vi "SRI8610C-DataFile Message Loop.vi"(7 "error in (no error)":errorcluster, 10 "Message Queues":T2) -> (0 "error out":errorcluster)   [LabVIEW 2020, in "SRI8610C-GasChromatograph.lvlib"]
uses:
  SRI8610C-GasChromatograph.lvlib
  support/Message Queue/All Message Queues.ctl
  support/Message Queue/Message Cluster.ctl
  SRI8160C/LabVIEW/Controls/SRI8610C-DataClusterV2.ctl
  SRI8160C/LabVIEW/Controls/SRI8610C-States-InitRun.ctl
  support/Message Queue/Enqueue Message (Single).vi
  support/Message Queue/Message Queue.lvlib
  Logging/Logging.lvlib
panel:
  out "Butane % Array":string[](array[string])
  out "GC Full Data Channels":T1[](array[typedef])
  out "Elapsed Time Since Last Update (sec)":dbl
  out "Numeric":i32
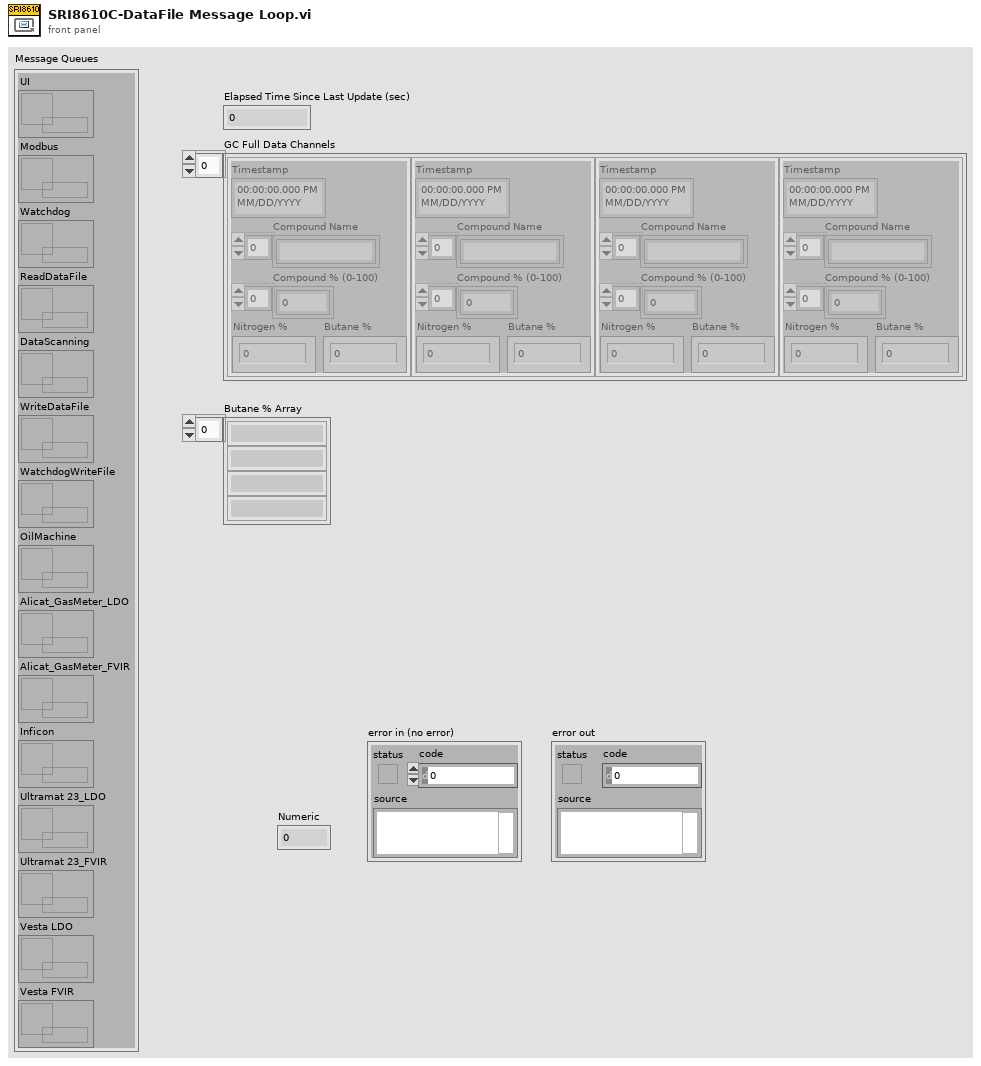
[diagram p1: front panel]
types:
  T1 = typedef "SRI8610C-DataClusterV2.ctl" = cluster{"Timestamp":timestamp, "Compound Name":string[], "Compound % (0-100)":dbl[], "Nitrogen %":dbl, "Butane %":dbl}
  T2 = typedef "Message Queue.lvlib/All Message Queues.ctl" = cluster{"UI":refnum<queue>, "Modbus":refnum<queue>, "Watchdog":refnum<queue>, "ReadDataFile":refnum<queue>, "DataScanning":refnum<queue>, "WriteDataFile":refnum<queue>, "WatchdogWriteFile":refnum<queue>, "OilMachine":refnum<queue>, "Alicat_GasMeter_LDO":refnum<queue>, "Inficon":refnum<queue>, "Ultramat 23_LDO":refnum<queue>, "Alicat_GasMeter_FVIR":refnum<queue>, "Ultramat 23_FVIR":refnum<queue>, "Vesta LDO":refnum<queue>, "Vesta FVIR":refnum<queue>}
  T3 = typedef "SRI8610C-States-InitRun.ctl" = enum16{"Initialize", "Run"}
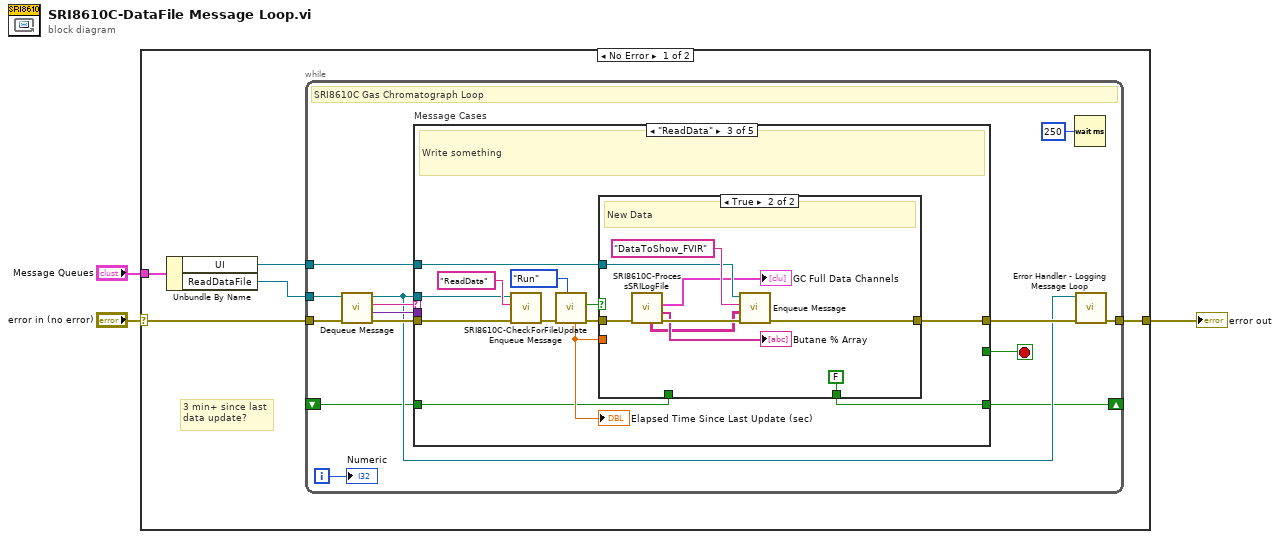
[diagram p0: block diagram]
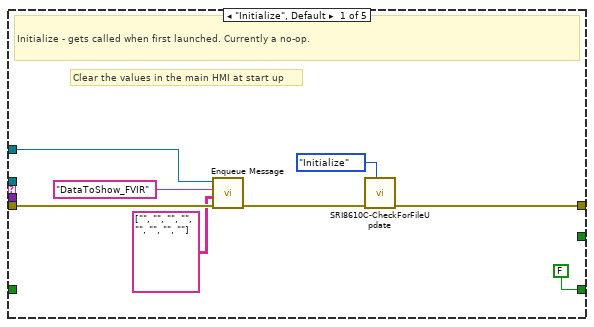
[diagram p2: hidden frame]
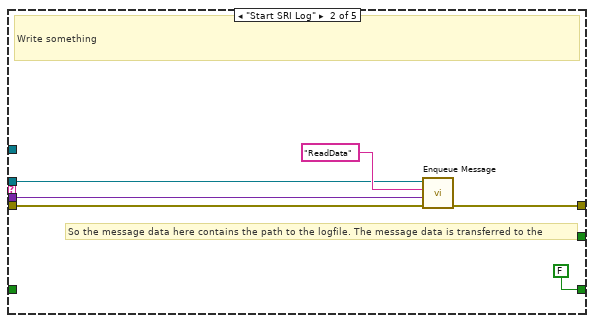
[diagram p3: hidden frame]
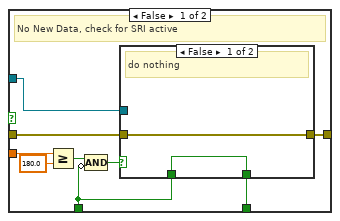
[diagram p4: hidden frame]
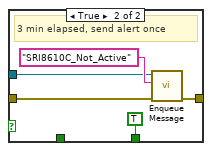
[diagram p5: hidden frame]
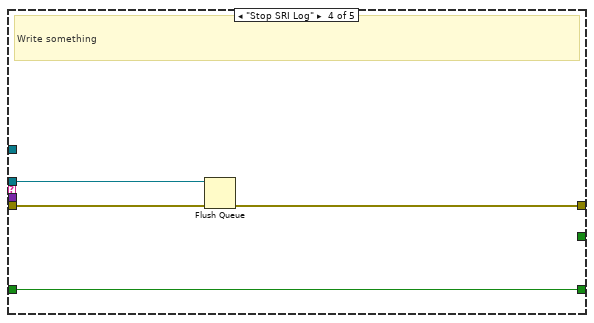
[diagram p6: hidden frame]
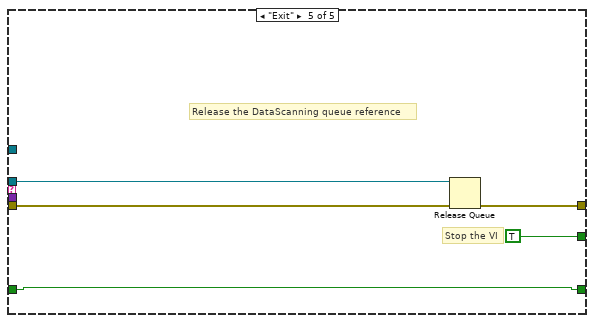
[diagram p7: hidden frame]
diagram:
  n1 = case shown="No Error" "error in (no error)" {
    selector: "error in (no error)" -> [w6 w82]
    tunnel: "Message Queues" -> [w8 _]
    tunnel: [w7 w82] -> w1
    frame No Error {
      # "3 min+ since last\ndata update?"
      n2 = Unbundle By Name(w8) -> ("UI"=w4:refnum<queue>, "ReadDataFile"=w5:refnum<queue>)
      n3 = while {
        tunnel: w5 -> [w17]
        tunnel: w6 -> [w21]
        tunnel: [w16] -> w7
        tunnel: w4 -> [w13]
        shift-right: [w9] -> _
        shift-left: _ -> [w10]
        i -> [w12]
        stop <- w22 stop-if-true
        # "SRI8610C Gas Chromatograph Loop"
        n4 = call "Dequeue Message.vi"("error in (no error)"=w21, "Message Queue"=w17) -> ("error out"=w20:errorcluster, "Message Data"=w18:variant, "Message"=w19:string, "dup Message Queue"=w14:refnum<queue>)  [unwired: 6 in]
        n5 = case "Message Cases" shown="\"ReadData\"" w19 {
          tunnel: w14 -> [_ w32 w44 w74 w80]
          tunnel: w20 -> [w29 w34 w46 w76 w78]
          tunnel: [w25 w36 w40 w75 w79] -> w15
          tunnel: [_ _ _ _ TRUE] -> w22
          tunnel: w18 -> [_ w33 _ _ _]
          tunnel: w13 -> [w30 _ w41 _ _]
          tunnel: w10 -> [_ _ w38 w73 w77]
          tunnel: [FALSE FALSE w37 w73 w77] -> w9
          frame "Initialize", Default {
            # "Clear the values in the main HMI at start up"
            # "Initialize - gets called when first launched. Currently a no-op."
            n6 = call-poly "Enqueue Message.vi"("error in (no error)"=w29, "Message Data"=string[][] [["", ""], ["", ""], ["", ""], ["", ""]], "Message"="DataToShow_FVIR", "Message Queue"=w30) -> ("error out"=w26:errorcluster)  [unwired: 6 in, 1 out]
            n7 = call "SRI8610C-CheckForFileUpdate.vi"("State"=SRI8610C-States-InitRun."Initialize", "error in"=w26) -> ("error out"=w25:errorcluster)  [unwired: 7 in, 2 out]
          }
          frame "Start SRI Log" {
            # "So the message data here contains the path to the logfile. The message data is transferred to the"
            # "Write something"
            n8 = call-poly "Enqueue Message.vi"("error in (no error)"=w34, "Message Data"=w33, "Message"="ReadData", "Message Queue"=w32) -> ("error out"=w36:errorcluster)  [unwired: 6 in, 1 out]
          }
          frame "ReadData" {
            # "Write something"
            n9 = call-poly "Enqueue Message.vi"("Message"="ReadData", "Message Queue"=w44) -> ()  [unwired: 8 in, 2 out]
            n10 = call "SRI8610C-CheckForFileUpdate.vi"("State"=SRI8610C-States-InitRun."Run", "error in"=w46) -> ("error out"=w43:errorcluster, "File Updated?"=w42:bool, "Elapsed Time Since Last Update (sec)"=w39:dbl)  [unwired: 7 in]
            "Elapsed Time Since Last Update (sec)" <- w39
            n11 = case shown="True" w42 {
              tunnel: w43 -> [w50 w72]
              tunnel: w41 -> [w54 w69]
              tunnel: [w52 w68] -> w40
              tunnel: w39 -> [w56 _]
              tunnel: w38 -> [w48 _]
              tunnel: [w49 FALSE] -> w37
              frame False {
                # "No New Data, check for SRI active"
                n12 = Greater Or Equal?(x=w56, y=180.0) -> (x >= y?=w53:bool)
                n13 = Compound Arithmetic op=AND(w53, invert w48) -> (w51:bool)
                n14 = case shown="False" w51 {
                  tunnel: w54 -> [_ w62]
                  tunnel: [w58 w61] -> w52
                  tunnel: w50 -> [w58 w60]
                  tunnel: [w57 TRUE] -> w49
                  tunnel: w48 -> [w57 _]
                  frame False {
                    # "do nothing"
                  }
                  frame True {
                    # "3 min elapsed, send alert once"
                    n15 = call-poly "Enqueue Message.vi"("error in (no error)"=w60, "Message"="SRI8610C_Not_Active", "Message Queue"=w62) -> ("error out"=w61:errorcluster)  [unwired: 7 in, 1 out]
                  }
                }
              }
              frame True {
                # "New Data"
                n16 = call "SRI8610C-ProcessSRILogFile.vi"("error in"=w72) -> ("error out"=w71:errorcluster, "Butane % Array"=→"Butane % Array":string[], "GC Full Data Channels"=→"GC Full Data Channels":T1[], "Formatted Data Output"=w64:string[][])  [unwired: 6 in, 1 out]
                n17 = call-poly "Enqueue Message.vi"("error in (no error)"=w71, "Message Data"=w64, "Message"="DataToShow_FVIR", "Message Queue"=w69) -> ("error out"=w68:errorcluster)  [unwired: 6 in, 1 out]
              }
            }
          }
          frame "Stop SRI Log" {
            # "Write something"
            n18 = Flush Queue(queue=w74, error in (no error)=w76) -> (error out=w75:errorcluster)  [unwired: 2 out]
          }
          frame "Exit" {
            # "Release the DataScanning queue reference"
            # "Stop the VI"
            n19 = Release Queue(queue=w80, error in (no error)=w78) -> (error out=w79:errorcluster)  [unwired: 1 in, 2 out]
          }
        }
        n20 = Wait (ms)(milliseconds to wait=u32 250) -> ()  [unwired: 1 out]
        n21 = call "Error Handler - Logging Message Loop.vi"("error in (no error)"=w15, "Message Queue"=w14) -> ("dup error in"=w16:errorcluster)  [unwired: 8 in, 1 out]
        "Numeric" <- w12
      }
    }
    frame Error {
    }
  }
  "error out" <- w1
